vi "ConvertV-F.vi"(8 "Test Name":string(combo)="WDW", 11 "Volt In":dbl format="%#_13g") -> (3 "Force Out":dbl)   [LabVIEW 2017]
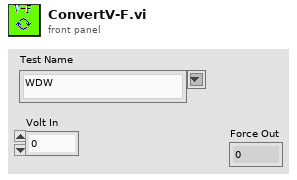
[diagram p1: front panel]
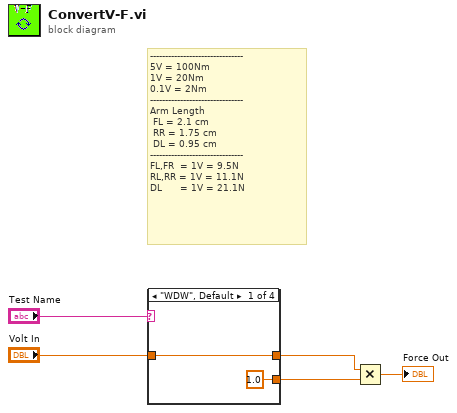
[diagram p0: block diagram]
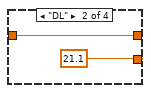
[diagram p2: hidden frame]
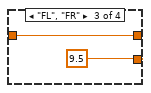
[diagram p3: hidden frame]
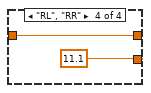
[diagram p4: hidden frame]
diagram:
  # "-------------------------------\n5V = 100Nm\n1V = 20Nm\n0.1V = 2Nm\n-------------------------------\nArm Length\n FL = 2.1 cm\n RR = 1.75 cm\n DL = 0.95 cm\n-------------------------------\nFL,FR  = 1V = 9.5N\nRL,RR = 1V = 11.1N\nDL      = 1V = 21.1N"
  n1 = case shown="\"WDW\", Default" "Test Name" {
    tunnel: [1.0 ("y") 21.1 ("y") 9.5 ("y") 11.1 ("y")] -> w4
    tunnel: "Volt In" -> [w7 w8 w10 w12]
    tunnel: [w7 w8 w10 w12] -> w1
    frame "WDW", Default {
    }
    frame "DL" {
    }
    frame "FL", "FR" {
    }
    frame "RL", "RR" {
    }
  }
  n2 = Multiply(x=w1, y=w4) -> (x*y=→"Force Out":dbl)
